vi "OPA.OrpheusHP.SetResource.vi"(8 "error in (no error)":errorcluster, 10 "Resource":T1, 11 "OPA.OrpheusHP in":refnum<class "OPA.OrpheusHP.lvclass">) -> (0 "error out":errorcluster, 3 "OPA.OrpheusHP out":refnum<class "OPA.OrpheusHP.lvclass">)   [LabVIEW 2019, in "OPA.OrpheusHP.lvclass"]
uses:
  OPA.OrpheusHP.lvclass
  Typedefs/Resource--Cluster.ctl
  E:/UPWORK/Laser Tool/Topas4PublicAPI/NET_SDK/Topas4Lib.dll
  Topas4PublicAPI/NET_SDK/Topas4Lib.dll
  OPA.OrpheusHP.lvclass/OPA.OrpheusHP.ctl
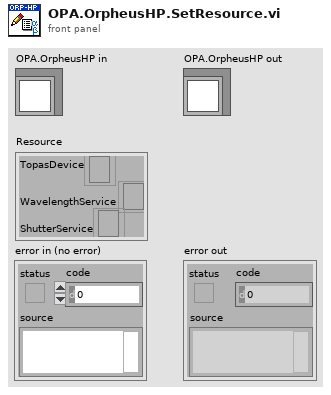
[diagram p1: front panel]
types:
  T1 = typedef "OPA.OrpheusHP.lvclass/Resource--Cluster.ctl" = cluster{"TopasDevice":refnum<k24>, "WavelengthService":refnum<k24>, "ShutterService":refnum<k24>}
  T2 = typedef "OPA.OrpheusHP.lvclass/PrivateData--Ref.ctl" = refnum<data-value>
  T3 = typedef "OPA.OrpheusHP.lvclass/PrivateData--Cluster.ctl" = cluster{"Resource":T1}
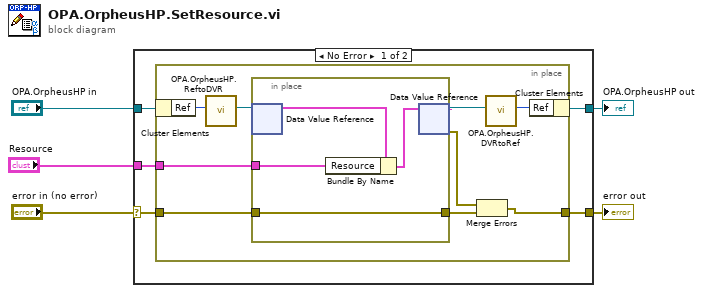
[diagram p0: block diagram]
diagram:
  n1 = case shown="No Error" "error in (no error)" {
    selector: "error in (no error)" -> [w7 w25]
    tunnel: [w6 w25] -> w4
    tunnel: [w9 w24] -> w2
    tunnel: "OPA.OrpheusHP in" -> [w10 w24]
    tunnel: "Resource" -> [w8 _]
    frame No Error {
      n2 = in-place {
        in-place-border: w8 -> [w16]
        in-place-border: w7 -> [w14]
        in-place-border: [w13] -> w6
        n3 = in-place-cluster #1(w10) -> ("Ref"=w18:u32)
        n4 = call "OPA.OrpheusHP.ReftoDVR.vi"("Ref"=w18) -> ("Ref"=w17:T2)  [unwired: 10 in]
        n5 = in-place {
          in-place-border: w16 -> [w22]
          in-place-border: [w20] -> w15
          in-place-border: w14 -> [w20]
          n6 = in-place-dvr #2(w17) -> (w23:T3)  [unwired: 1 out]
          n7 = Bundle By Name(cluster=w23, "Resource"=w22) -> (w21:T3)
          n8 = in-place-dvr #2(w21) -> (w12:T2, w11:errorcluster)
        }
        n9 = Merge Errors(w11, w15) -> (w13:errorcluster)
        n10 = call "OPA.OrpheusHP.DVRtoRef.vi"("Ref"=w12) -> ("Ref"=w19:u32)  [unwired: 10 in]
        n11 = in-place-cluster #1("Ref"=w19) -> (w9:refnum<class "OPA.OrpheusHP.lvclass">)
      }
    }
    frame Error {
    }
  }
  "error out" <- w4
  "OPA.OrpheusHP out" <- w2
